vi "pt_andrei.vi"() -> ()   [LabVIEW 2015]
uses:
  <vilib>/imath/engines/lvmath/Plug In/_Char/NIMS_CH_character datatype.ctl
  <vilib>/imath/engines/lvmath2/RunTimeEngine/Managers/WorkSpace/UID Generator.vi
  <vilib>/imath/engines/lvmath/Plug In/_Char/NIMS_CH_String to Character Array.vi
  <vilib>/imath/engines/lvmath/Plug In/_Char/NIMS_CH_Character RV to String.vi
  <vilib>/imath/engines/lvmath2/RunTimeEngine/BuiltInFunctions/fopen/NIMS_fopen(Str).vi
  <vilib>/imath/engines/lvmath2/RunTimeSupport/NIMS_Get Scalar_w Error.vi
  <instcachedir>/0/NIMS_Get Scalar_w Error_412A576220DD41E68C0A524E94A2DE79.lvgen/NIMS_Get Scalar_w Error_412A576220DD41E68C0A524E94A2DE79_010.vi
  <vilib>/imathl/engines/lvmath/Functions/Error Handling/Create Error.vi
  <vilib>/imath/engines/lvmath2/RunTimeEngine/BuiltInFunctions/fscanf/NIMS_[DBLM,I32]=fscanf.vi
  <vilib>/imath/engines/lvmath2/RunTimeEngine/BuiltInFunctions/transpose/NIMS_transpose(GM).vi
  <instcachedir>/0/NIMS_transpose(GM)_822C4B39CC3F4B34B360A85316D387F1.lvgen/NIMS_transpose(GM)_822C4B39CC3F4B34B360A85316D387F1_004.vi
  <vilib>/imath/engines/lvmath2/RunTimeEngine/BuiltInFunctions/view_image/NIMS_view_image.vi
  <vilib>/imath/engines/lvmath2/RunTimeEngine/BuiltInFunctions/fclose/NIMS_fclose(fid).vi
  <vilib>/imath/engines/lvmath2/RunTimeEngine/ErrorHandling/NIMS_Finalize Error.vi
panel:
  in  "String 2":string
  in  "String":string
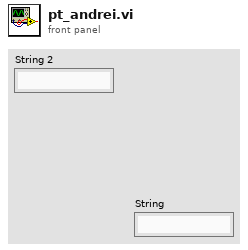
[diagram p1: front panel]
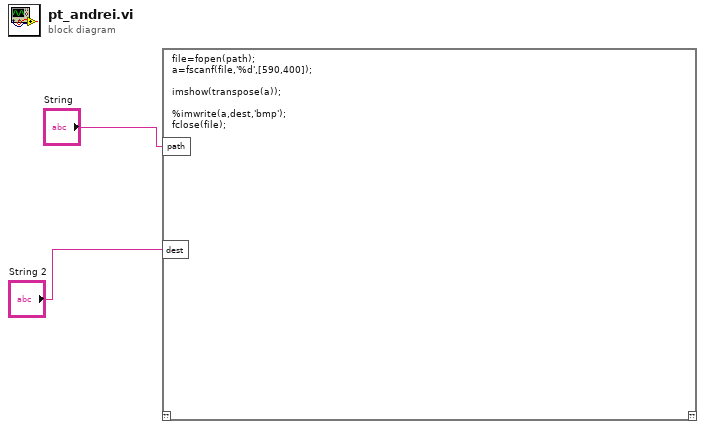
[diagram p0: block diagram]
diagram:
  n1 = mathscript code="file=fopen(path);\na=fscanf(file,'%d',[590,400]);\n\nimshow(transpose(a));\n\n%imwrite(a,dest,'bmp');\nfclose(file);"("path"="String", "dest"="String 2") -> ()  [unwired: 1 in, 1 out]
